vi "Sensirion SHT25 - VISA write user register.vi"(8 "Error In":errorcluster, 10 "user register (in)":u8 format="%08b", 11 "VISA in":refnum<visa-resource-name>) -> (0 "Error Out":errorcluster, 1 "user register (out)":u8 format="%08b", 3 "VISA out":refnum<visa-resource-name>)   [LabVIEW 2012]
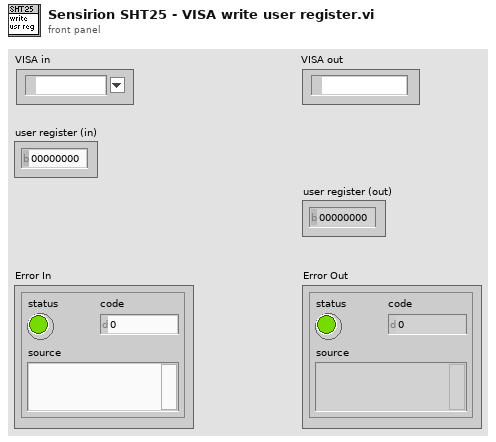
[diagram p1: front panel]
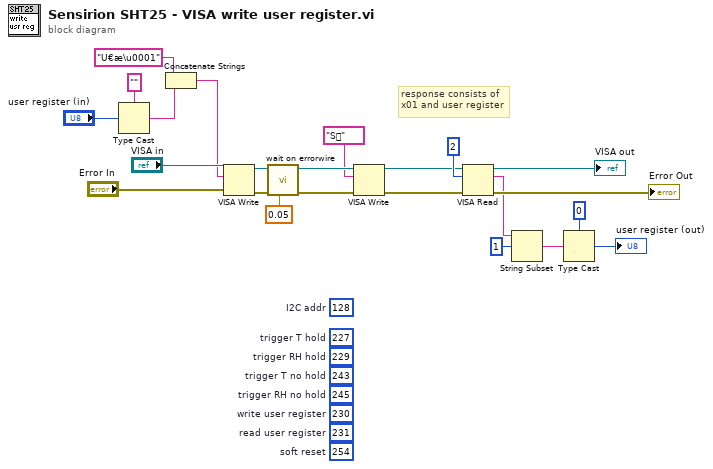
[diagram p0: block diagram]
diagram:
  (unwired) u8 254  # soft reset
  (unwired) u8 231  # read user register
  (unwired) u8 230  # write user register
  (unwired) u8 245  # trigger RH no hold
  (unwired) u8 243  # trigger T no hold
  (unwired) u8 229  # trigger RH hold
  (unwired) u8 128  # I2C addr
  (unwired) u8 227  # trigger T hold
  # "response consists of\nx01 and user register"
  n1 = Type Cast(type="" ("element"), x="user register (in)") -> (*(type *) &x=w1:string)
  n2 = Concatenate Strings("U€æ\u0001", w1) -> (w4:string)
  n3 = VISA Write(VISA resource name="VISA in", write buffer=w4, error in (no error)="Error In") -> (VISA resource name out=w15:refnum<visa-resource-name>, error out=w19:errorcluster)  [unwired: 1 out]
  n4 = call "wait on errorwire.vi"("Delay Time (s)"=0.05, "error in (no error)"=w19) -> ("error out"=w14:errorcluster)  [unwired: 9 in]
  n5 = VISA Write(VISA resource name=w15, write buffer="S", error in (no error)=w14) -> (VISA resource name out=w12:refnum<visa-resource-name>, error out=w13:errorcluster)  [unwired: 1 out]
  n6 = VISA Read(VISA resource name=w12, byte count=u32 2, error in (no error)=w13) -> (VISA resource name out=→"VISA out":refnum<visa-resource-name>, read buffer=w10:string, error out=→"Error Out":errorcluster)  [unwired: 1 out]
  n7 = String Subset(string=w10, offset (0)=1) -> (substring=w8:string)  [unwired: 1 in]
  n8 = Type Cast(type=u8 0 ("element"), x=w8) -> (*(type *) &x=→"user register (out)":u8)
